vi "H5set_free_list_limits.vi"(6 "error in (no error)":errorcluster, 9 "Memory Limits":T1={"Global Regular Limit"=-1, "List Regular Limit"=-1, "Global Array Limit"=-1, "List Array Limit"=-1, "Global Block Limit"=-1, "List Block Limit"=-1}) -> (0 "error out":errorcluster)   [LabVIEW 2017]
doc: "Sets free-list size limits."
uses:
  <vilib>/UPVI/lvhdf5/hdf5.dll
panel:
  # "LVHDF5 Toolkit\nCopyright (c) 2005-2013 by Jason D. Sommerville\nCopyright (c) 2014 by UPVI, LLC.\n\nThis use and distribution of this file is governed by the terms found in \nLICENSE.txt distributed with this toolkit and installed at\n <user.lib>\\_lvhdf5\\LICENSE.txt"
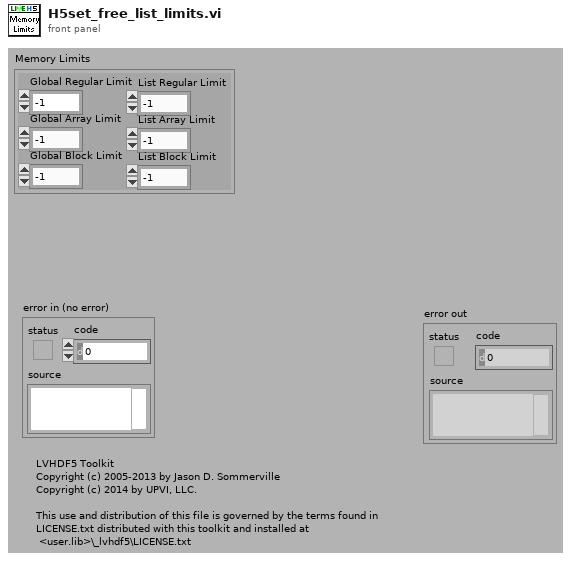
[diagram p1: front panel]
types:
  T1 = cluster{"Global Regular Limit":i32, "List Regular Limit":i32, "Global Array Limit":i32, "List Array Limit":i32, "Global Block Limit":i32, "List Block Limit":i32}
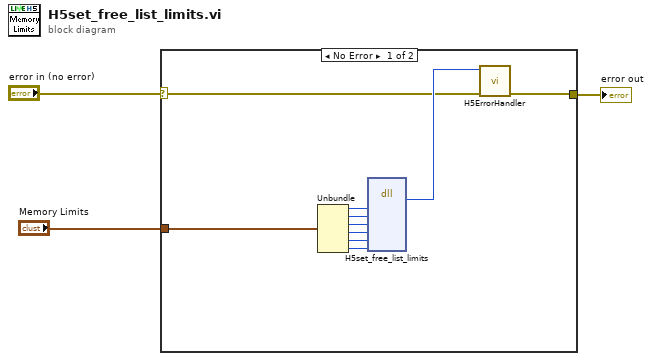
[diagram p0: block diagram]
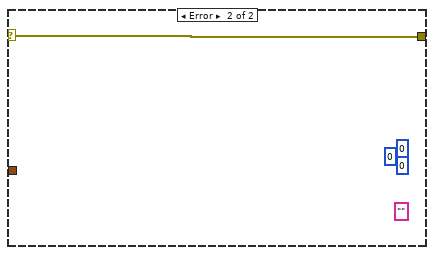
[diagram p2: hidden frame]
diagram:
  n1 = case shown="No Error" "error in (no error)" {
    selector: "error in (no error)" -> [w12 w14]
    tunnel: [w11 w14] -> w2
    tunnel: "Memory Limits" -> [w10 _]
    frame No Error {
      n2 = Unbundle(w10) -> ("Global Regular Limit"=w9:i32, "List Regular Limit"=w8:i32, "Global Array Limit"=w7:i32, "List Array Limit"=w6:i32, "Global Block Limit"=w5:i32, "List Block Limit"=w4:i32)
      n3 = dll-call lib="C:/Program Files/National Instruments/LabVIEW 2017/vi.lib/UPVI/lvhdf5/hdf5.dll" fn="H5set_free_list_limits"("reg_global_lim"=w9, "reg_list_lim"=w8, "arr_global_lim"=w7, "arr_list_lim"=w6, "blk_global_lim"=w5, "blk_list_lim"=w4) -> (w13:i32)  [unwired: 9 in, 2 out]
      n4 = call <vilib>:"H5ErrorHandler.vi"("error in (no error)"=w12, "herr_t"=w13) -> ("error out"=w11:errorcluster)  [unwired: 3 in, 4 out]
    }
    frame Error {
      (unwired) ""
      (unwired) u32 0 ("relnum")
      (unwired) u32 0 ("minnum")
      (unwired) u32 0 ("majnum")
    }
  }
  "error out" <- w2
